vi "Trapezoidal Motion Profile.vi"(7 "Reset?":bool, 10 "Distance":dbl) -> (2 "Throttle Out":sgl, 4 "Finished?":bool)   [LabVIEW 2015]
uses:
  Robot Code/Robot Global Data.vi
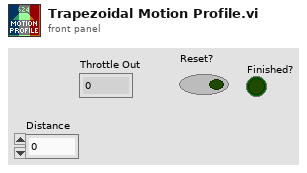
[diagram p1: front panel]
types:
  T1 = typedef "Dashboard Control Data.ctl" = cluster{"Encoder Control":T2, "Steer PID output":cluster{"output high":dbl, "output low":dbl}, " Steer PID gains":cluster{"proportional gain (Kc)":dbl, "integral time (Ti, min)":dbl, "derivative time (Td, min)":dbl}, "Drivetrain Settings":T3, "Vision Packet":T4, "Dashboard Drivetrain Command":T5, "Info/Command Cluster":T7, "Ball Vision Packet":T8, "Intake Presets":T10, "Intake Encoder Control":T12, "Climb Presets":T13, "Goal Output Range":cluster{"output high":dbl, "output low":dbl}, "Enabled Systems":T14, "Auton Presets":T15, "Pressure M":dbl, "Pressure B":dbl, "Vision Timeout":dbl, "Auto-Shift":T16, "Catapult Setpoints":T17}
  T2 = typedef "Encoder Control.ctl" = cluster{"Right Tick Constant":dbl, "Left Tick Constant":dbl, "Reset?":bool, "Y Dist":cluster{"PID gains":cluster{"proportional gain (Kc)":dbl, "integral time (Ti, min)":dbl, "derivative time (Td, min)":dbl}}, "Y Stop Thresh":dbl, "Y Stop Speed":dbl}
  T3 = typedef "Drivetrain Settings.ctl" = cluster{"Gyro Tolerance":dbl, "Throttle Ramp (ms)":dbl, "Kv":dbl, "Ka":dbl, "Feed Forward P":dbl, "Feed Forward D":dbl, "Goal Vision PID gains":cluster{"proportional gain (Kc)":dbl, "integral time (Ti, min)":dbl, "derivative time (Td, min)":dbl}, "Goal Detection Window":dbl, "Creep Rate":dbl, "Vision Throttle Threshold":dbl, "Min Turn Output":dbl, "Left Batter Angle":dbl, "Right Batter Angle":dbl}
  T4 = typedef "Goal Vision Packet.ctl" = cluster{"Distance":dbl, "Center X":dbl, "Center Y":dbl, "Found Target?":bool, "Robot Center":dbl, "Angle":dbl}
  T5 = typedef "Dashboard Drivetrain Command.ctl" = cluster{"Drivetrain Vision":T6}
  T6 = typedef "Drivetrain Vision.ctl" = cluster{"Goal Window":dbl, "Ball Window":dbl}
  T7 = typedef "Ball Tracking Command Cluster.ctl" = cluster{"Distance to Ball":dbl, "Desired Angle":dbl, "Command":enum16{"Turn to Ball", "Turn to Angle", "Get Distance"}, "Pixels from Center":dbl}
  T8 = typedef "Ball Vision Packet.ctl" = cluster{"Ball Detected?":bool, "Distance to Ball":dbl, "Desired Angle":dbl, "Pixels from Center":dbl, "Tracking mode":T9}
  T9 = typedef "Tracking Mode.ctl" = enum16{"Turn to Ball", "Turn to Angle"}
  T10 = typedef "Intake Presets.ctl" = cluster{"Intake Speed":dbl, "Outake Speed":dbl, "Angle Speed":dbl, "Angle Tolerance":dbl, "Encoder Scale":dbl, "Load Height":dbl, "Output Range":T11, "MaxCurrent":dbl, "Idle Height":dbl, "Max Height":dbl, "Reset Encoders?":bool, "PID gains":cluster{"proportional gain (Kc)":dbl, "integral time (Ti, min)":dbl, "derivative time (Td, min)":dbl}, "Drop Low Height ":dbl, "Rotation Power Max/Min":dbl}
  T11 = typedef "Drivetrain Output Range.ctl" = cluster{"output high":dbl, "output low":dbl}
  T12 = typedef "IntakeEcoderControl.ctl" = cluster{"Arm Tick Constant":dbl, "Reset?":bool, "Y Dist":cluster{"PID gains":cluster{"proportional gain (Kc)":dbl, "integral time (Ti, min)":dbl, "derivative time (Td, min)":dbl}}, "Y Stop Thresh":dbl, "Y Stop Speed":dbl}
  T13 = typedef "Climb Presets.ctl" = cluster{"Pull Power":dbl, "Extend Power":dbl}
  T14 = typedef "Enabled Systems.ctl" = cluster{"Shoot":bool, "Intake":bool, "DT":bool, "Gyro":bool, "100ms":bool, "US":bool}
  T15 = typedef "Autonomous Presets.ctl" = cluster{"Pitch Limit":dbl, "Roll Limit":dbl, "Start Position":dbl, "Cross Position":dbl}
  T16 = typedef "Auto Shift Cluster.ctl" = cluster{"Delay":dbl, "Speed Thresh":dbl, "Upshift Accel":dbl, "Upshift Throttle":dbl, "Upshift Throttle Accel":dbl, "Downshift Throttle":dbl, "Downshift Throttle Accel":dbl, "Pressure Threshold":dbl}
  T17 = typedef "Catapult Presets.ctl" = cluster{"Intake Danger Height":dbl, "Ball Security Delay ":dbl, "High PSI Minimum":dbl, "Shot Finish Delay":dbl, "Low PSI Minimum":dbl, "Idle Ball Security Wait ":dbl}
  T18 = typedef "Encoder Values Super Cluster.ctl" = cluster{"Left Encoder":T19, "Right Encoder":T19}
  T19 = typedef "Encoder Values.ctl" = cluster{"Distance":dbl, "Speed":dbl, "Ticks":dbl}
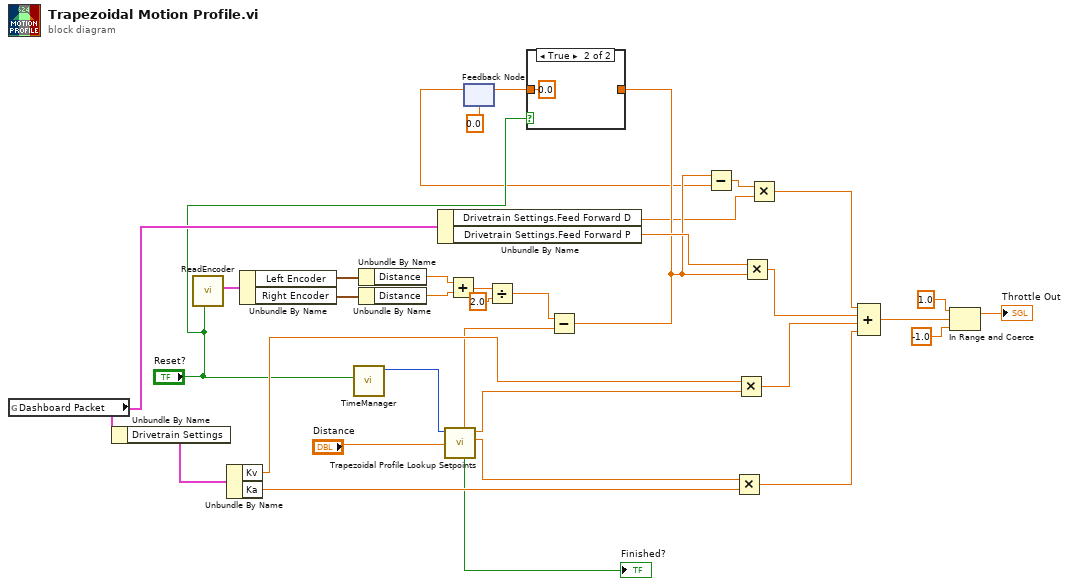
[diagram p0: block diagram]
diagram:
  n1 = global read "Robot Global Data.vi" "Dashboard Packet"() -> (w14:T1)
  n2 = Unbundle By Name(w14) -> ("Drivetrain Settings"=w27:T3)
  n3 = call "ReadEncoder.vi"("Reset?"="Reset?") -> ("Quick Use Cluster"=w24:T18)  [unwired: 10 in]
  n4 = Unbundle By Name(w27) -> ("Kv"=w26:dbl, "Ka"=w25:dbl)
  n5 = Unbundle By Name(w24) -> ("Left Encoder"=w23:T19, "Right Encoder"=w22:T19)
  n6 = call "TimeManager.vi"("Reset?"="Reset?") -> ("Time Since Reset"=w34:u32)  [unwired: 9 in, 1 out]
  n7 = Unbundle By Name(w23) -> ("Distance"=w21:dbl)
  n8 = Unbundle By Name(w22) -> ("Distance"=w20:dbl)
  n9 = Unbundle By Name(w14) -> ("Drivetrain Settings.Feed Forward D"=w6:dbl, "Drivetrain Settings.Feed Forward P"=w13:dbl)
  n10 = call "Trapezoidal Profile Lookup Setpoints.vi"("Total Distance"="Distance", "Current Time"=w34) -> ("Acceleration"=w30:sgl, "Velocity"=w29:sgl, "Profile Completed?"=→"Finished?":bool, "Projected Current Distance"=w16:dbl)  [unwired: 6 in]
  n11 = Add(x=w21, y=w20) -> (x+y=w19:dbl)
  n12 = feedback #1(0.0) -> (w8:dbl)
  n13 = Divide(x=w19, y=2.0) -> (x/y=w15:dbl)
  n14 = Subtract(x=w15, y=w16) -> (x-y=w9:dbl)
  n15 = case shown="True" "Reset?" {
    tunnel: [w35 0.0] -> w11
    tunnel: w9 -> [w35 _]
    frame False {
    }
    frame True {
    }
  }
  n16 = feedback-in #1(w11) -> ()
  n17 = Subtract(x=w9, y=w8) -> (x-y=w7:dbl)
  n18 = Multiply(x=w30, y=w25) -> (x*y=w2:dbl)
  n19 = Multiply(x=w26, y=w29) -> (x*y=w3:dbl)
  n20 = Multiply(x=w13, y=w9) -> (x*y=w4:dbl)
  n21 = Multiply(x=w7, y=w6) -> (x*y=w5:dbl)
  n22 = Compound Arithmetic op=ADD(w5, w4, w3, w2) -> (w1:dbl)
  n23 = In Range and Coerce(upper limit=sgl 1.0, x=w1, lower limit=sgl -1.0) -> (coerced(x)=→"Throttle Out":dbl)  [unwired: 1 out]
